vi "Write Instrument Ini file.vi"(8 "error in (no error)":errorcluster, 11 "User List":string[](array[string])) -> (0 "error out":errorcluster)   [LabVIEW 2020, in "Test Framework.lvclass"]
doc: "Reads the instrument ini file and outputs the instrument and reference choices"
uses:
  Test Framework.lvclass
  <vilib>/Utility/config.llb/Write Key (String).vi
  <vilib>/Utility/config.llb/NI_LVConfig.lvlib
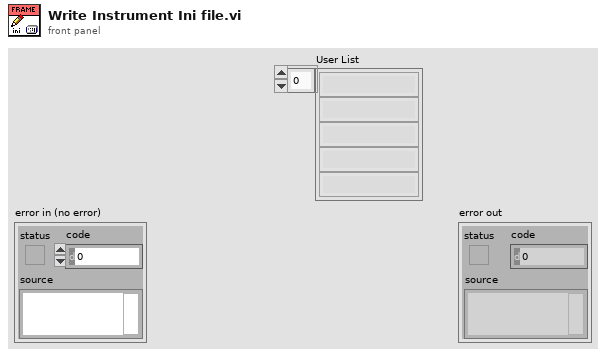
[diagram p1: front panel]
types:
  T1 = typedef "NI_LVConfig.lvlib/Config Data RefNum.ctl" = refnum<k1>
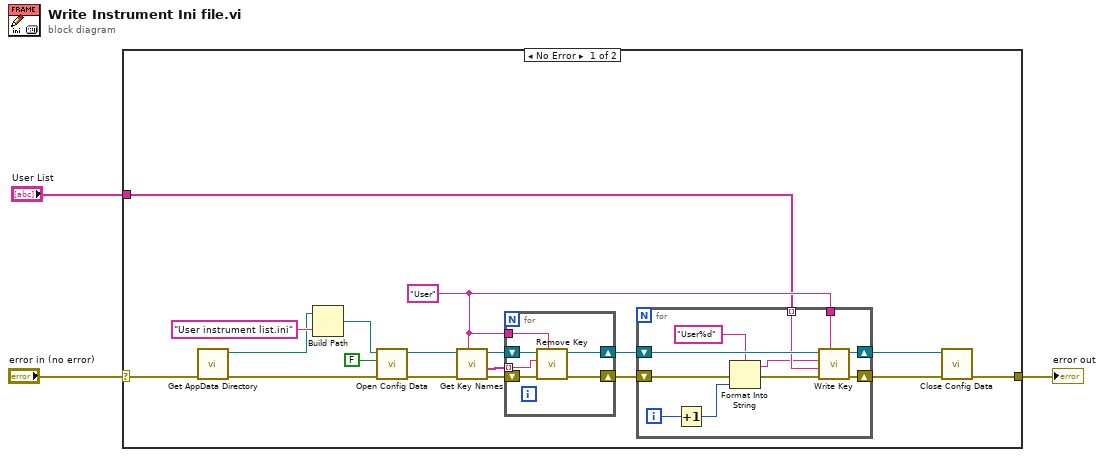
[diagram p0: block diagram]
diagram:
  n1 = case shown="No Error" "error in (no error)" {
    selector: "error in (no error)" -> [w5 w39]
    tunnel: [w7 w39] -> w2
    tunnel: "User List" -> [w11 _]
    frame No Error {
      w12 = "User" ("section")
      n2 = call "Get AppData Directory.vi"("Error In"=w5) -> ("Error Out"=w4:errorcluster, "Folder path"=w6:path)  [unwired: 8 in, 1 out]
      n3 = Build Path(base path=w6, name or relative path="User instrument list.ini") -> (appended path=w20:path)
      n4 = call <vilib>:"Open Config Data.vi"("error in (no error)"=w4, "create file if necessary (T)"=FALSE, "configuration file path"=w20) -> ("error out"=w18:errorcluster, "refnum"=w17:T1)  [unwired: 6 in, 1 out]
      n5 = call <vilib>:"Get Key Names.vi"("section"=w12, "error in (no error)"=w18, "refnum"=w17) -> ("error out"=w16:errorcluster, "key names"=w15:string[], "refnum out"=w14:T1)  [unwired: 5 in, 1 out]
      n6 = for {
        shift-right: [w37] -> w13
        shift-left: w16 -> [w38]
        tunnel: w15 -> [w33] mode=indexing
        tunnel: w12 -> [w35]
        shift-right: [w34] -> w9
        shift-left: w14 -> [w36]
        n7 = call <vilib>:"Remove Key.vi"("section"=w35, "error in (no error)"=w38, "key"=w33, "refnum"=w36) -> ("error out"=w37:errorcluster, "refnum out"=w34:T1)  [unwired: 5 in, 1 out]
      }
      n8 = for {
        shift-right: [w32] -> w10
        shift-left: w13 -> [w23]
        tunnel: w12 -> [w31]
        tunnel: w11 -> [w28] mode=indexing
        shift-right: [w29] -> w8
        shift-left: w9 -> [w30]
        i -> [w26]
        n9 = Increment(x=w26) -> (x+1=w25:i32)
        n10 = Format Into String(format string="User%d", error in=w23, w25) -> (resulting string=w24:string, error out=w22:errorcluster)  [unwired: 1 in]
        n11 = call-poly <vilib>:"Write Key.vi"("section"=w31, "error in (no error)"=w22, "value"=w28, "key"=w24, "refnum"=w30) -> ("error out"=w32:errorcluster, "refnum out"=w29:T1)  [unwired: 4 in, 1 out]
      }
      n12 = call <vilib>:"Close Config Data.vi"("error in (no error)"=w10, "refnum"=w8) -> ("error out"=w7:errorcluster)  [unwired: 8 in, 1 out]
    }
    frame Error {
    }
  }
  "error out" <- w2
